vi "起摆摆角变换-子.vi"(3 "摆角输入":dbl) -> (0 "循环条件":bool, 1 "摆角输出":dbl)   [LabVIEW 2015]
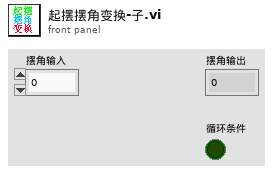
[diagram p1: front panel]
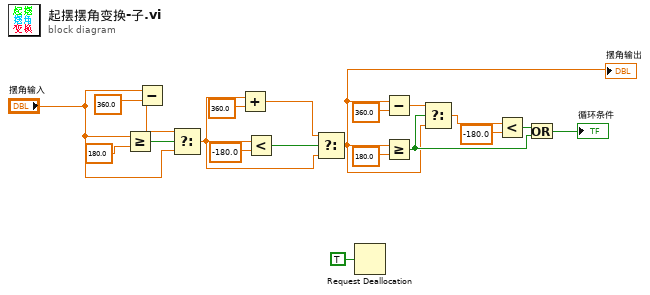
[diagram p0: block diagram]
diagram:
  n1 = Greater Or Equal?(x="摆角输入", y=180.0) -> (x >= y?=w19:bool)
  n2 = Subtract(x="摆角输入", y=360.0) -> (x-y=w17:dbl)
  n3 = Select(t=w17, s=w19, f="摆角输入") -> (s? t:f=w12:dbl)
  n4 = Add(x=w12, y=360.0) -> (x+y=w14:dbl)
  n5 = Less?(x=w12, y=-180.0) -> (x < y?=w15:bool)
  n6 = Select(t=w14, s=w15, f=w12) -> (s? t:f=w2:dbl)
  "摆角输出" <- w2
  n7 = Request Deallocation(TRUE ("标志")) -> ()
  n8 = Subtract(x=w2, y=360.0) -> (x-y=w9:dbl)
  n9 = Greater Or Equal?(x=w2, y=180.0) -> (x >= y?=w5:bool)
  n10 = Select(t=w9, s=w5, f=w2) -> (s? t:f=w7:dbl)
  n11 = Less?(x=w7, y=-180.0) -> (x < y?=w6:bool)
  n12 = Or(x=w6, y=w5) -> (x .or. y?=→"循环条件":bool)
